vi "Send to CS.vi"(8 "error in (no error)":errorcluster, 10 "String to write":string, 11 "PCS in":refnum<class "PCS.lvclass">) -> (0 "error out":errorcluster, 3 "PCS out":refnum<class "PCS.lvclass">)   [LabVIEW 2019, in "PCS.lvclass"]
uses:
  Lib.llb/PCS.lvclass
  Lib.llb/QCS.lvclass
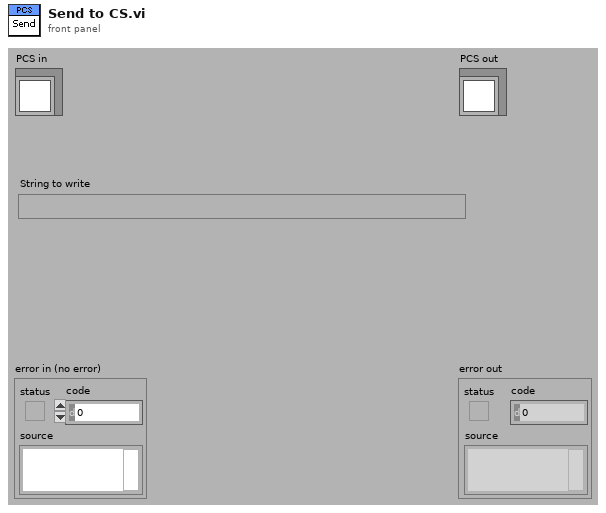
[diagram p1: front panel]
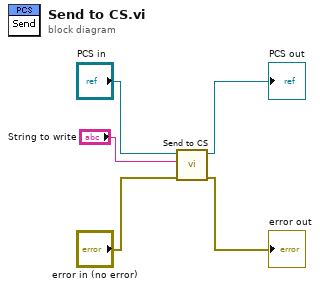
[diagram p0: block diagram]
diagram:
  n1 = call-parent "Send to CS.vi"("error in (no error)"="error in (no error)", "String to write"="String to write", "QCS in"="PCS in") -> ("error out"=→"error out":errorcluster, "QCS out"=→"PCS out":refnum<class "PCS.lvclass">)  [unwired: 7 in]
